vi "Exit.vi"(7 "Exit Notifier":refnum<notifier>, 8 "error in (no error)":errorcluster, 10 "UI Queue":refnum<queue>, 11 "Message Queue":refnum<queue>) -> (0 "error out":errorcluster)   [LabVIEW 2014, in "Logger.lvlib"]
uses:
  Logger.lvlib
  support/Message Queue/Message Queue.lvlib
  support/Message Queue/Message Cluster.ctl
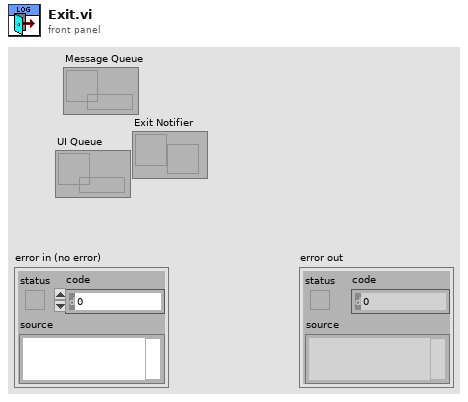
[diagram p1: front panel]
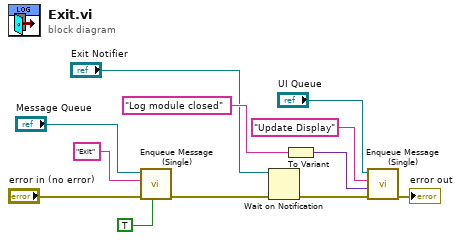
[diagram p0: block diagram]
diagram:
  n1 = call "Enqueue Message (Single).vi"("Priority Message? (F)"=TRUE, "error in (no error)"="error in (no error)", "Message"="Exit", "Message Queue"="Message Queue") -> ("error out"=w9:errorcluster)  [unwired: 6 in, 1 out]
  n2 = Wait on Notification(notifier="Exit Notifier", error in (no error)=w9) -> (error out=w8:errorcluster)  [unwired: 2 in, 3 out]
  n3 = To Variant(anything="Log module closed" ("Message")) -> (Variant=w4:variant)
  n4 = call "Enqueue Message (Single).vi"("error in (no error)"=w8, "Message Data"=w4, "Message"="Update Display", "Message Queue"="UI Queue") -> ("error out"=→"error out":errorcluster)  [unwired: 6 in, 1 out]
